vi "Load Cell Test.vi"() -> ()   [LabVIEW 2018]
uses:
  <vilib>/Utility/error.llb/DialogType.ctl
  <vilib>/Platform/TimedLoop/XDataNode/timing_clust.ctl
  <vilib>/Platform/TimedLoop/XDataNode/nitl_modes.ctl
  <vilib>/Platform/TimedLoop/XDataNode/wakeup.ctl
  <vilib>/DAQmx/read.llb/DAQmx Read (Analog DBL 1Chan 1Samp).vi
  <vilib>/DAQmx/configure/timing.llb/DAQmx Timing (Implicit).vi
  <vilib>/DAQmx/miscellaneous.llb/DAQmx Fill In Error Info.vi
  <vilib>/platform/TimedLoop/XDataNode/XDataNode.xnode
  <vilib>/Platform/TimedLoop/XDataNode/XDNodeRunTimeDep.lvlib
panel:
  out "Waveform Chart":dbl(graph)
  out "data":dbl format="%0.2f"
  in  "Stop":bool
  out "Iteration Duration (uS)":i64
  in  "Sample Rate":dbl=1000.0
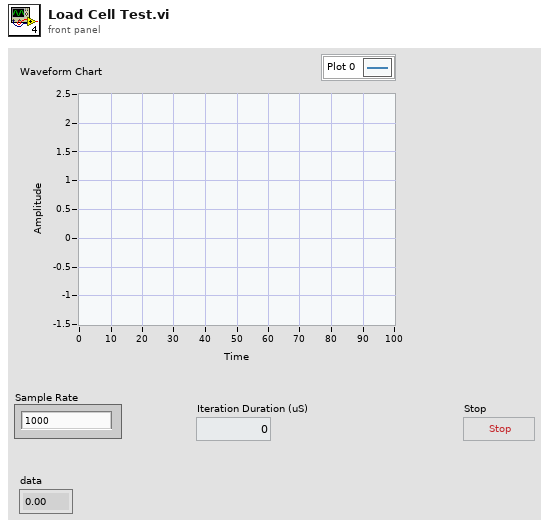
[diagram p1: front panel]
types:
  T1 = typedef "DialogType.ctl" = u16
  T2 = typedef "XDNodeRunTimeDep.lvlib/timing_clust.ctl" = cluster{"Expected End [f-1]":u64, "Actual End [f-1]":u64, "Finished Late? [f-1]":bool, "Expected End [i-1]":u64, "Actual End [i-1]":u64, "Finished Late? [i-1]":bool, "Expected Start [i]":u64, "Actual Start [i]":u64, "Expected Start [f]":u64, "Actual Start [f]":u64, "Source Name":string, "Structure Name":string, "Period":i64, "Deadline":i64, "Offset":i64, "Start":i64, "Priority":i32, "Timeout":i32, "Mode":T3, "Wakeup Reason":T4, "Error":errorcluster, "Source Type":string, "Secondary Source Type":string, "Global End Time":u64, "Global Start Time":u64, "Frame Duration":u64, "Iteration Duration":u64, "Assigned CPU":i32, "I/O Scan Engine Mode":u32}
  T3 = typedef "XDNodeRunTimeDep.lvlib/nitl_modes.ctl" = enum32{"No Change", "Process missed periods, maintain original phase", "Discard missed periods, maintain original phase", "Process missed periods, ignore original phase", "Discard missed periods, ignore original phase"}
  T4 = typedef "XDNodeRunTimeDep.lvlib/wakeup.ctl" = enum32{"Normal", "Aborted", "Asynchronous wakeup", "Timing source error", "Timed loop error", "Timeout"}
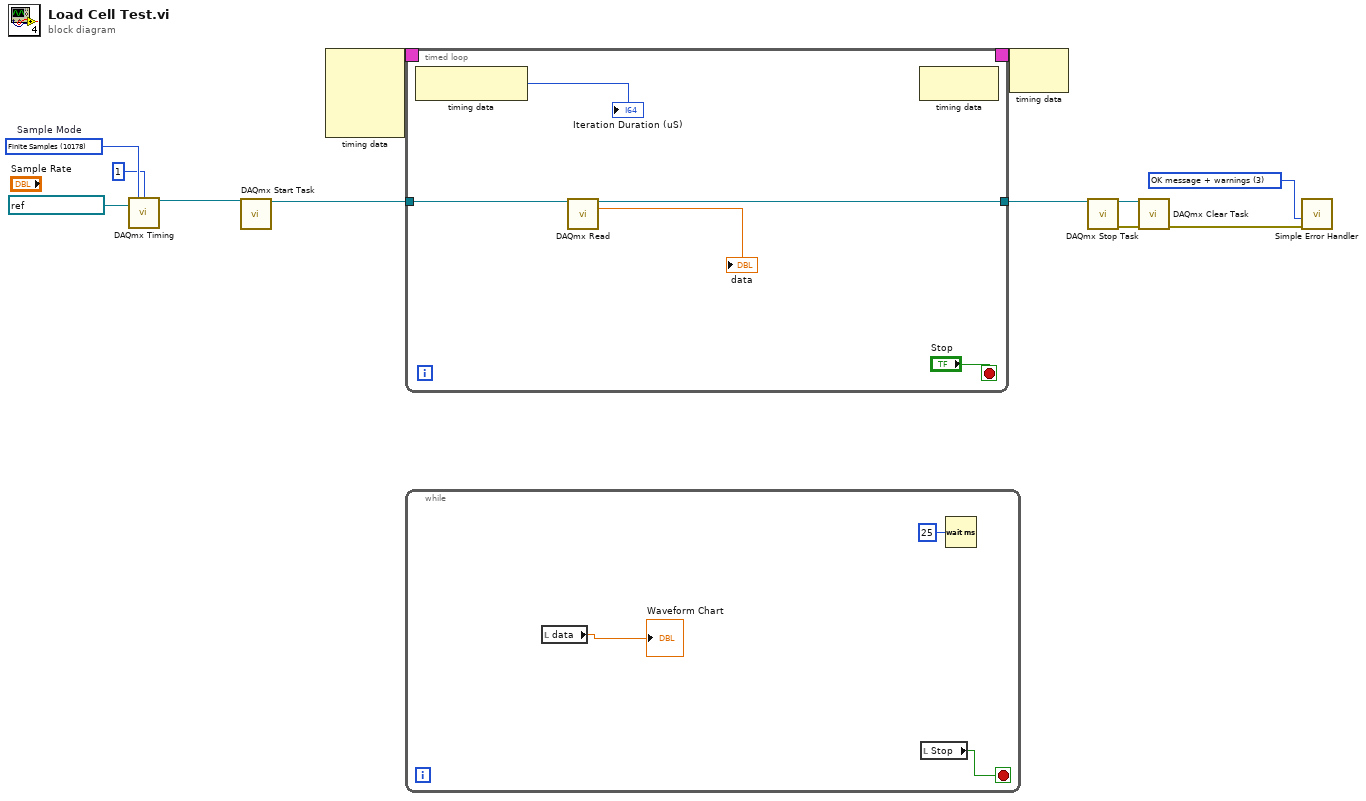
[diagram p0: block diagram]
diagram:
  w3 = T1 3 items=["no dialog", "OK message", "continue or stop message", "OK message + warnings", "continue/stop + warnings"] ("type of dialog (OK msg:1)")
  w12 = 10178 items=["Finite Samples"=10178, "Continuous Samples"=10123, "Hardware Timed Single Point"=12522]  # Sample Mode
  n1 = call-poly <vilib>:"DAQmx Timing.vi"("task/channels in"=refnum<k21> "Futek 844206", "sample mode"=w12, "samples per channel"=1) -> ("task out"=w10:refnum<k21>)  [unwired: 11 in, 1 out]
  n2 = call <vilib>:"DAQmx Start Task.vi"("task/channels in"=w10) -> ("task out"=w7:refnum<k21>)  [unwired: 13 in, 1 out]
  n3 = node-c288() -> (w9:T2)  [unwired: 4 in]
  n4 = timed-loop {
    timing: w9 -> [_]
    timing-out: [_] -> w8
    tunnel: w7 -> [w17]
    tunnel: [w15] -> w2
    stop <- "Stop" stop-if-true
    n5 = node-c288() -> (→"Iteration Duration (uS)":i64)  [unwired: 1 in]
    n6 = call-poly <vilib>:"DAQmx Read.vi"("task/channels in"=w17) -> ("task out"=w15:refnum<k21>, "data"=→"data":dbl)  [unwired: 12 in, 1 out]
    n7 = node-c288() -> ()  [unwired: 1 in, 1 out]
  }
  n8 = while {
    stop <- w21 stop-if-true
    n9 = local read "data"() -> (→"Waveform Chart":dbl)
    n10 = local read "Stop"() -> (w21:bool)
    n11 = Wait (ms)(milliseconds to wait=u32 25) -> ()  [unwired: 1 out]
  }
  n12 = node-c288(w8) -> ()  [unwired: 1 out]
  n13 = call <vilib>:"DAQmx Stop Task.vi"("task/channels in"=w2) -> ("task out"=w5:refnum<k21>, "error out"=w4:errorcluster)  [unwired: 13 in]
  n14 = call <vilib>:"DAQmx Clear Task.vi"("task in"=w5, "error in"=w4) -> ("error out"=w6:errorcluster)  [unwired: 13 in]
  n15 = call <vilib>:"Simple Error Handler.vi"("type of dialog (OK msg:1)"=w3, "error in (no error)"=w6) -> ()  [unwired: 3 in, 5 out]
